vi "Mathcad Prime cmd.vi"(6 "Mathcad Prime cmds":T3, 8 "error in (no error)":errorcluster, 11 "DesignRequest":T1) -> (0 "error out":errorcluster, 2 "Mathcad Output":T2, 3 "DesignRequest out":T1)   [LabVIEW 2015]
uses:
  Folders.ctl
  Mathcad Prime cmds.ctl
  Variable cluster.ctl
  Design Request.ctl
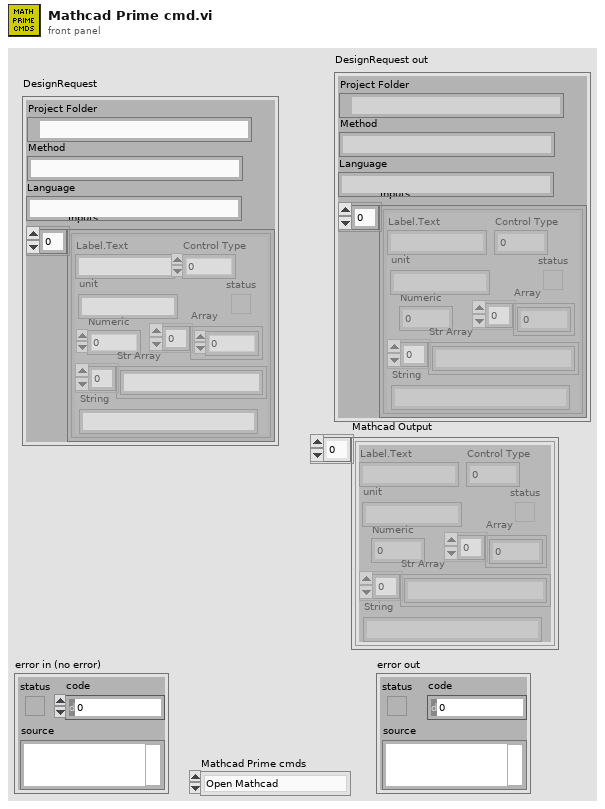
[diagram p1: front panel]
types:
  T1 = typedef "Design Request.ctl" = cluster{"Project Folder":path, "Method":string, "Inputs":T2, "Language":string}
  T2 = typedef "Variable cluster.ctl" = cluster{"Label.Text":string, "Control Type":u32, "Numeric":dbl, "Array":dbl[], "status":bool, "Str Array":string[], "String":string, "unit":string}[]
  T3 = typedef "Mathcad Prime cmds.ctl" = enum16{"Open Mathcad", "Open Worksheet", "Send Inputs", "Read Results", "Quit Mathcad"}
  T4 = typedef "Folders.ctl" = enum16{"DesignTool", "RequestedDesigns", "CompletedDesigns"}
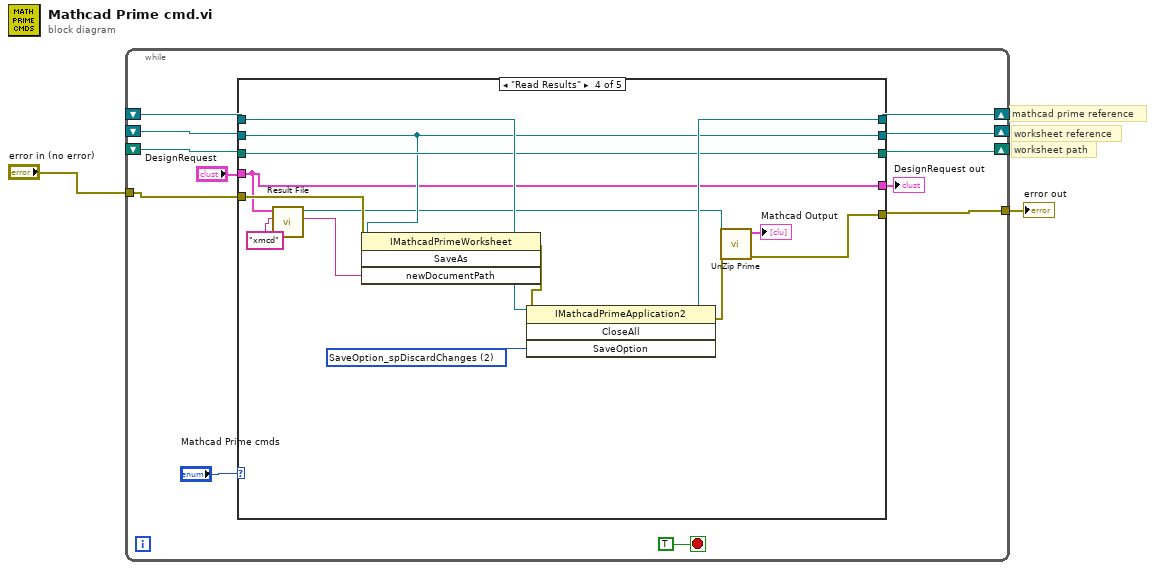
[diagram p0: block diagram]
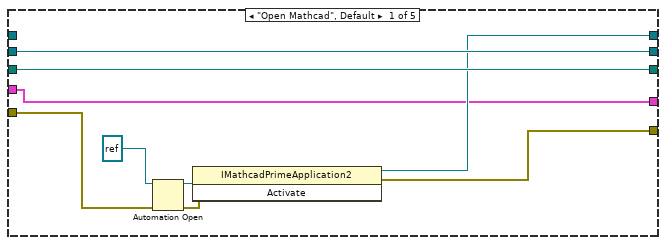
[diagram p2: hidden frame]
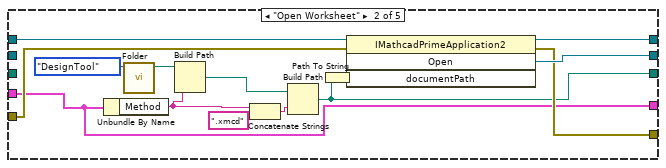
[diagram p3: hidden frame]
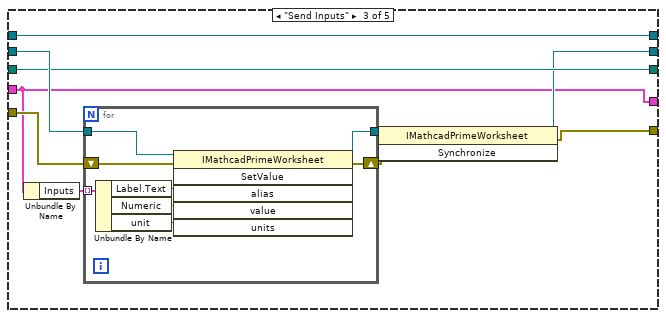
[diagram p4: hidden frame]
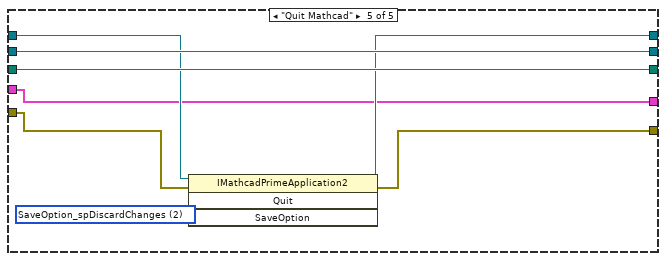
[diagram p5: hidden frame]
diagram:
  # "worksheet path"
  # "worksheet reference"
  # "mathcad prime reference"
  n1 = while {
    tunnel: "error in (no error)" -> [w13]
    tunnel: [w12] -> w1
    shift-right: [w11] -> _
    shift-left: _ -> [w10]
    shift-right: [w8] -> _
    shift-left: _ -> [w7]
    shift-right: [w5] -> _
    shift-left: _ -> [w6]
    stop <- TRUE stop-if-true
    n2 = case shown="\"Read Results\"" "Mathcad Prime cmds" {
      tunnel: w13 -> [w22 w36 w45 w62 w72]
      tunnel: [w20 w29 w42 w65 w71] -> w12
      tunnel: [w17 w30 w40 w66 w73] -> w11
      tunnel: w10 -> [_ w37 w40 w68 w74]
      tunnel: "DesignRequest" -> [w15 w24 w38 w56 w70]
      tunnel: [w19 w31 w39 w63 w77] -> w8
      tunnel: w7 -> [w19 _ w46 w63 w77]
      tunnel: [w18 w28 w41 w64 w76] -> w5
      tunnel: w6 -> [w18 _ w41 w64 w76]
      tunnel: [w15 w24 w38 w56 w70] -> w3
      frame "Open Mathcad", Default {
        n3 = Automation Open(error in (no error)=w22, Automation Refnum=refnum<k7> refnum ("MathcadPrime.IMathcadPrimeApplication2")) -> (Automation Refnum=w23:refnum<k7>, error out=w21:errorcluster)  [unwired: 2 in]
        n4 = invoke class="IMathcadPrimeApplication2" method="Activate"(reference=w23, error in=w21) -> (reference out=w17:refnum<k7>, error out=w20:errorcluster)  [unwired: 1 in, 1 out]
      }
      frame "Open Worksheet" {
        n5 = Unbundle By Name(w24) -> ("Method"=w25:string)
        n6 = call "Folder.vi"("Folders"=Folders."DesignTool") -> ("FolderPath"=w27:path)  [unwired: 9 in, 1 out]
        n7 = Build Path(base path=w27, name or relative path=w25) -> (appended path=w26:path)
        n8 = Concatenate Strings(w25, ".xmcd" ("string")) -> (w34:string)
        n9 = Build Path(base path=w26, name or relative path=w34) -> (appended path=w28:path)
        n10 = Path To String(path=w28) -> (string=w32:string)
        n11 = invoke class="IMathcadPrimeApplication2" method="Open"(reference=w37, error in=w36, "documentPath"=w32) -> (reference out=w30:refnum<k7>, error out=w29:errorcluster, "Open"=w31:refnum<k7>)  [unwired: 1 in, 1 out]
      }
      frame "Send Inputs" {
        n12 = Unbundle By Name(w38) -> ("Inputs"=w47:T2)
        n13 = for {
          tunnel: w47 -> [w55] mode=indexing
          tunnel: w46 -> [w51]
          tunnel: [w50] -> w44
          shift-right: [w49] -> w43
          shift-left: w45 -> [w48]
          n14 = Unbundle By Name(w55) -> ("Label.Text"=w53:string, "Numeric"=w54:dbl, "unit"=w52:string)
          n15 = invoke class="IMathcadPrimeWorksheet" method="SetValue"(reference=w51, error in=w48, "alias"=w53, "value"=w54, "units"=w52) -> (reference out=w50:refnum<k7>, error out=w49:errorcluster)  [unwired: 1 in, 4 out]
        }
        n16 = invoke class="IMathcadPrimeWorksheet" method="Synchronize"(reference=w44, error in=w43) -> (reference out=w39:refnum<k7>, error out=w42:errorcluster)  [unwired: 1 in, 1 out]
      }
      frame "Read Results" {
        w67 = 2 items=["SaveOption_spSaveChanges", "SaveOption_spPromptToSaveChanges", "SaveOption_spDiscardChanges"] ("SaveOption")
        n17 = call "Result File.vi"("File Type"="xmcd" ("string"), "DesignRequest"=w56) -> ("File string"=w58:string, "File path"=w57:path)  [unwired: 8 in]
        n18 = invoke class="IMathcadPrimeWorksheet" method="SaveAs"(reference=w63, error in=w62, "newDocumentPath"=w58) -> (error out=w61:errorcluster)  [unwired: 1 in, 3 out]
        n19 = invoke class="IMathcadPrimeApplication2" method="CloseAll"(reference=w68, error in=w61, "SaveOption"=w67) -> (reference out=w66:refnum<k7>, error out=w69:errorcluster)  [unwired: 1 in, 2 out]
        n20 = call "UnZip Prime.vi"("error in"=w69, "Path"=w57) -> ("error out"=w65:errorcluster, "Variable Clusters out"=→"Mathcad Output":T2)  [unwired: 8 in]
      }
      frame "Quit Mathcad" {
        w75 = 2 items=["SaveOption_spSaveChanges", "SaveOption_spPromptToSaveChanges", "SaveOption_spDiscardChanges"] ("SaveOption")
        n21 = invoke class="IMathcadPrimeApplication2" method="Quit"(reference=w74, error in=w72, "SaveOption"=w75) -> (reference out=w73:refnum<k7>, error out=w71:errorcluster)  [unwired: 1 in, 2 out]
      }
    }
    "DesignRequest out" <- w3
  }
  "error out" <- w1
